vi "PostSnapshot.vi"(8 "error in (no error)":errorcluster, 11 "LogManager in":refnum<class "LogManager.lvclass">) -> (0 "error out":errorcluster, 3 "LogManager out":refnum<class "LogManager.lvclass">)   [LabVIEW 2026, in "Lumberjack.lvlib" / "LogManager.lvclass"]
doc: "Build the current Snapshot (global threshold from resolvedConfig, and the array of appender enqueuers from the registry) and post it to the shared Notifier via Send Notification. Callers read this snapshot non-destructively on the hot path. Called after any change to the threshold or appender set: initial launch, register, unregister, and threshold change. The LogManager is the sole poster of the Notifier (SRS-LMBR-052, design 2.1)."
uses:
  LogManager.lvclass
  TypeDefs/Snapshot.ctl
  TypeDefs/Severity.ctl
  <vilib>/ActorFramework/Message Enqueuer/Message Enqueuer.lvclass
  LogManager.lvclass/LogManager.ctl
  Lumberjack.lvlib
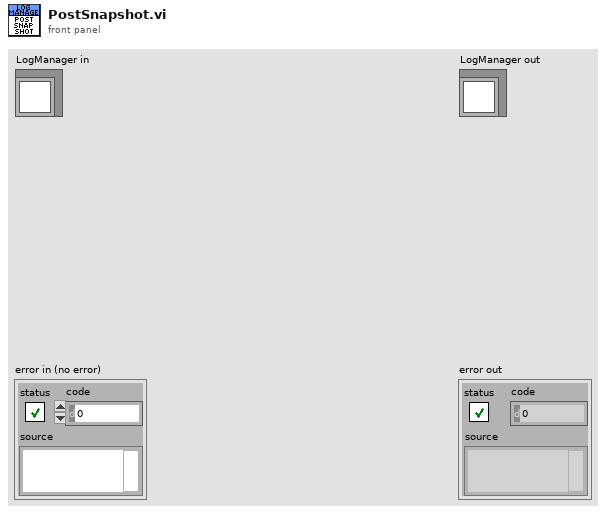
[diagram p1: front panel]
types:
  T1 = typedef "Lumberjack.lvlib/Snapshot.ctl" = cluster{"globalThreshold":T2, "appenderEnqueuers":cluster{"id":string, "enqueuer":refnum<class "Message Enqueuer.lvclass">}[]}
  T2 = typedef "Lumberjack.lvlib/Severity.ctl" = enum16{"OFF", "FATAL", "ERROR", "WARN", "INFO", "DEBUG", "TRACE", "ALL"}
  T3 = typedef "Lumberjack.lvlib/RegistryEntry.ctl" = cluster{"id":string, "enqueuer":refnum<class "Message Enqueuer.lvclass">}
  T4 = cluster{"id":string, "enqueuer":refnum<class "Message Enqueuer.lvclass">}
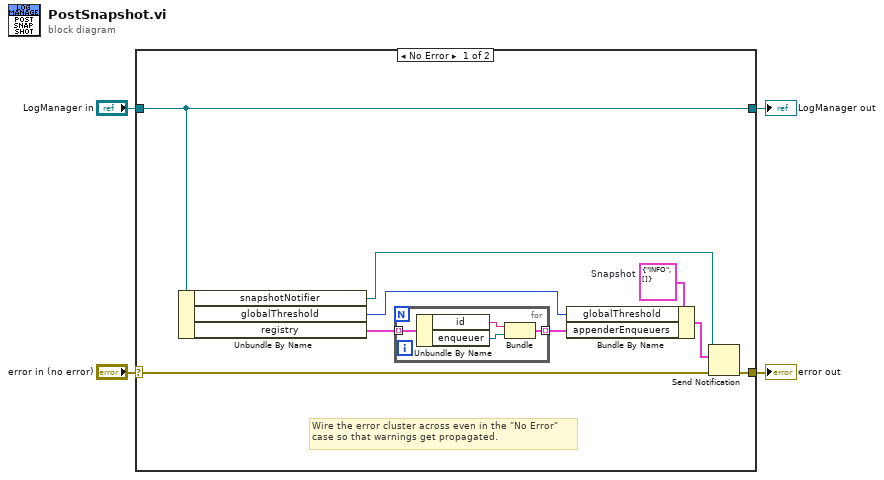
[diagram p0: block diagram]
diagram:
  n1 = case shown="No Error" "error in (no error)" {
    selector: "error in (no error)" -> [w10 w19]
    tunnel: [w9 w19] -> w3
    tunnel: [w13 w18] -> w1
    tunnel: "LogManager in" -> [w13 w18]
    frame No Error {
      w7 = T1 {"globalThreshold"=enum."INFO", "appenderEnqueuers"=[]}  # Snapshot
      # "Wire the error cluster across even in the \"No Error\"\ncase so that warnings get propagated."
      n2 = Unbundle By Name(w13) -> ("snapshotNotifier"=w6:refnum<notifier>, "globalThreshold"=w5:T2, "registry"=w12:T3[])
      n3 = for {
        tunnel: w12 -> [w17] mode=indexing
        tunnel: [w14] -> w11 mode=indexing
        n4 = Unbundle By Name(w17) -> ("id"=w16:string, "enqueuer"=w15:refnum<class "Message Enqueuer.lvclass">)
        n5 = Bundle("id"=w16, "enqueuer"=w15) -> (w14:T4)  [unwired: 1 in]
      }
      n6 = Bundle By Name(cluster=w7, "globalThreshold"=w5, "appenderEnqueuers"=w11) -> (w8:T1)
      n7 = Send Notification(notification=w8, notifier=w6, error in (no error)=w10) -> (error out=w9:errorcluster)  [unwired: 1 out]
    }
    frame Error {
    }
  }
  "error out" <- w3
  "LogManager out" <- w1
